vi "FTW-Subscriber-Subscribe.vi"(5 "Addresses":string, 9 "Buffer Depth (1 element)":i32=1, 11 "error in":errorcluster) -> (4 "FTW-Subscription Out":refnum<class "FTW-Subscriber.lvclass">, 6 "Subscriber Registration":refnum<event-registration>, 15 "error out":errorcluster)   [LabVIEW 2013, in "FTW-Subscriber.lvclass"]
uses:
  FTW-Subscriber.lvclass
  Message/Base/FTW-Message.lvclass
  Message/Lossy/FTW-Message-Lossy.lvclass
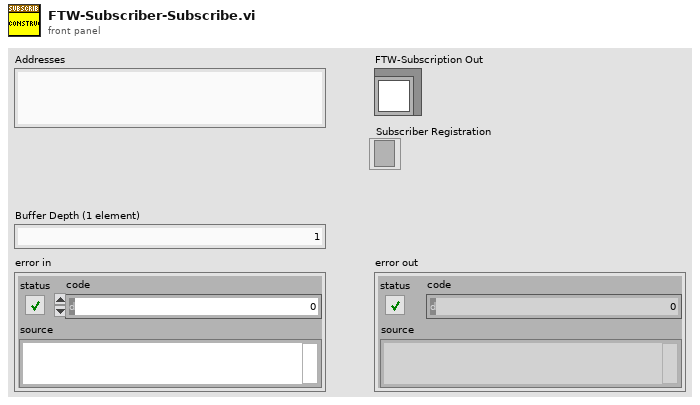
[diagram p1: front panel]
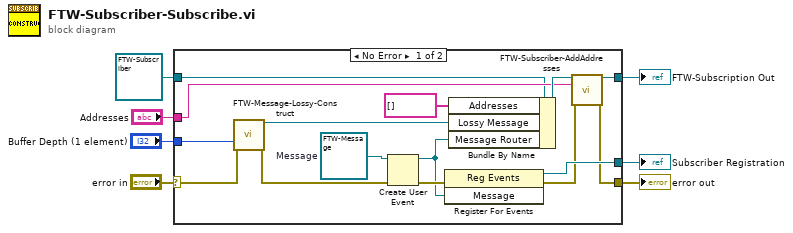
[diagram p0: block diagram]
diagram:
  n1 = case shown="No Error" "error in" {
    selector: "error in" -> [w17 w24]
    tunnel: [w16 w24] -> w6
    tunnel: [w18 w23] -> w5
    tunnel: [w21 _] -> w2
    tunnel: "Addresses" -> [w14 _]
    tunnel: refnum<class "FTW-Subscriber.lvclass"> refnum ("LVmsg_Router.lvclass") -> [w11 w23]
    tunnel: "Buffer Depth (1 element)" -> [w8 _]
    frame No Error {
      w20 = refnum<class "FTW-Message.lvclass"> refnum  # Message
      n2 = call "FTW-Message-Lossy-Construct.vi"("max queue size (1)"=w8, "error in"=w17) -> ("FTW-Message-Lossy"=w9:refnum<class "FTW-Message-Lossy.lvclass">, "error out"=w10:errorcluster)  [unwired: 12 in]
      n3 = Create User Event(user event datatype=w20, error in=w10) -> (user event=w12:refnum<user-event>, error out=w19:errorcluster)
      n4 = register-events(error in=w19, w12) -> (reference out=w21:refnum<event-registration>, error out=w15:errorcluster)  [unwired: 1 in]
      n5 = Bundle By Name(cluster=w11, "Addresses"=string[] [], "Lossy Message"=w9, "Message Router"=w12) -> (w22:refnum<class "FTW-Subscriber.lvclass">)
      n6 = call "FTW-Subscriber-AddAddresses.vi"("FTW-Subscription In"=w22, "Addresses"=w14, "error in"=w15) -> ("FTW-Subscription Out"=w18:refnum<class "FTW-Subscriber.lvclass">, "error out"=w16:errorcluster)  [unwired: 11 in]
    }
    frame Error {
    }
  }
  "FTW-Subscription Out" <- w5
  "error out" <- w6
  "Subscriber Registration" <- w2
